vi "Test Filtering.vi"(8 "error in (no error)":errorcluster) -> (0 "error out":errorcluster)   [LabVIEW 2020]
uses:
  a02d23f6-73dd-4d4c-9f99-b180725647c3.vi
  533fd5d0-9135-456a-82c4-707cf62dfcc0.vi
  b2c899c7-82cb-45de-b54c-0f6bbd6c2dd8.vi
  1299700a-be9c-46a6-9b80-003b6c5b12f7.vi
  808b52e7-524e-4250-8ad6-d26fecc8b44a.vi
  3354226a-df3f-4c2f-8e3d-1360450e1ad8.vi
  205459d0-1598-4474-bf47-9f69c46f8ece.vi
  486e4e40-c95f-4fac-875a-f5feb60e7227.vi
  533fd5d0-9135-456a-82c4-707cf62dfcc0.vi/44d2b068-fa24-42c4-b7ce-acd781796053.vi
  533fd5d0-9135-456a-82c4-707cf62dfcc0.vi/f7e9a4a8-169a-4713-a4c5-2a646feda0be.vi
  533fd5d0-9135-456a-82c4-707cf62dfcc0.vi/4f5c7ada-fea6-4248-8bb4-58b212ee00ca.vi
  b2c899c7-82cb-45de-b54c-0f6bbd6c2dd8.vi/d1fab985-9124-480e-b8bc-aa5377d2de92.vi
  1299700a-be9c-46a6-9b80-003b6c5b12f7.vi/b73cea84-e472-4b9c-965d-660adbe74b39.vi
  808b52e7-524e-4250-8ad6-d26fecc8b44a.vi/683d2099-e00c-4551-b026-3c1073bcb77e.vi
  3354226a-df3f-4c2f-8e3d-1360450e1ad8.vi/eacad6df-34c9-4c9e-8205-0119b8e818d4.vi
  205459d0-1598-4474-bf47-9f69c46f8ece.vi/8ef18e61-07fd-42c8-9af4-61308265cf71.vi
  205459d0-1598-4474-bf47-9f69c46f8ece.vi/8f8b69a5-3137-4430-b83e-41fe2cca619b.vi
  205459d0-1598-4474-bf47-9f69c46f8ece.vi/2a0a81ed-9654-4ad9-8980-5ddc2610bcd7.vi
  205459d0-1598-4474-bf47-9f69c46f8ece.vi/17cfa5ab-349d-4170-9ba1-b7281e37bcf7.vi
  486e4e40-c95f-4fac-875a-f5feb60e7227.vi/6ddd74e0-5d25-4d4f-89c3-674211749c19.vi
  486e4e40-c95f-4fac-875a-f5feb60e7227.vi/1dcbab8f-0ca2-4569-972e-ee80beb773d1.vi
  486e4e40-c95f-4fac-875a-f5feb60e7227.vi/9005e1d8-42db-4b2c-8892-941e6a8eeacc.vi
  486e4e40-c95f-4fac-875a-f5feb60e7227.vi/8a9e105b-ea02-4efd-9282-f92cd78db5c5.vi
  b2c899c7-82cb-45de-b54c-0f6bbd6c2dd8.vi/d1fab985-9124-480e-b8bc-aa5377d2de92.vi/eacad6df-34c9-4c9e-8205-0119b8e818d4.vi
  486e4e40-c95f-4fac-875a-f5feb60e7227.vi/8a9e105b-ea02-4efd-9282-f92cd78db5c5.vi/8aece534-05e1-49aa-ae6d-ba885b1b7e2e.vi
  <vilib>/addons/_JKI Toolkits/Caraya/classes/Assert/Assert Equal Value and Type_Variant.vi
  <vilib>/addons/_JKI Toolkits/Caraya/classes/Assert/Assert Equal Value_Variant.vi
  <vilib>/Comparison/Equal/Equal Functor/Equal Functor.lvclass
  <vilib>/addons/_JKI Toolkits/Caraya/classes/Test/Test.lvclass
  <vilib>/addons/_JKI Toolkits/Caraya/classes/Assert/Assert.lvclass
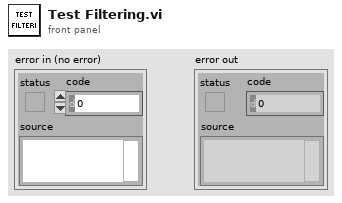
[diagram p1: front panel]
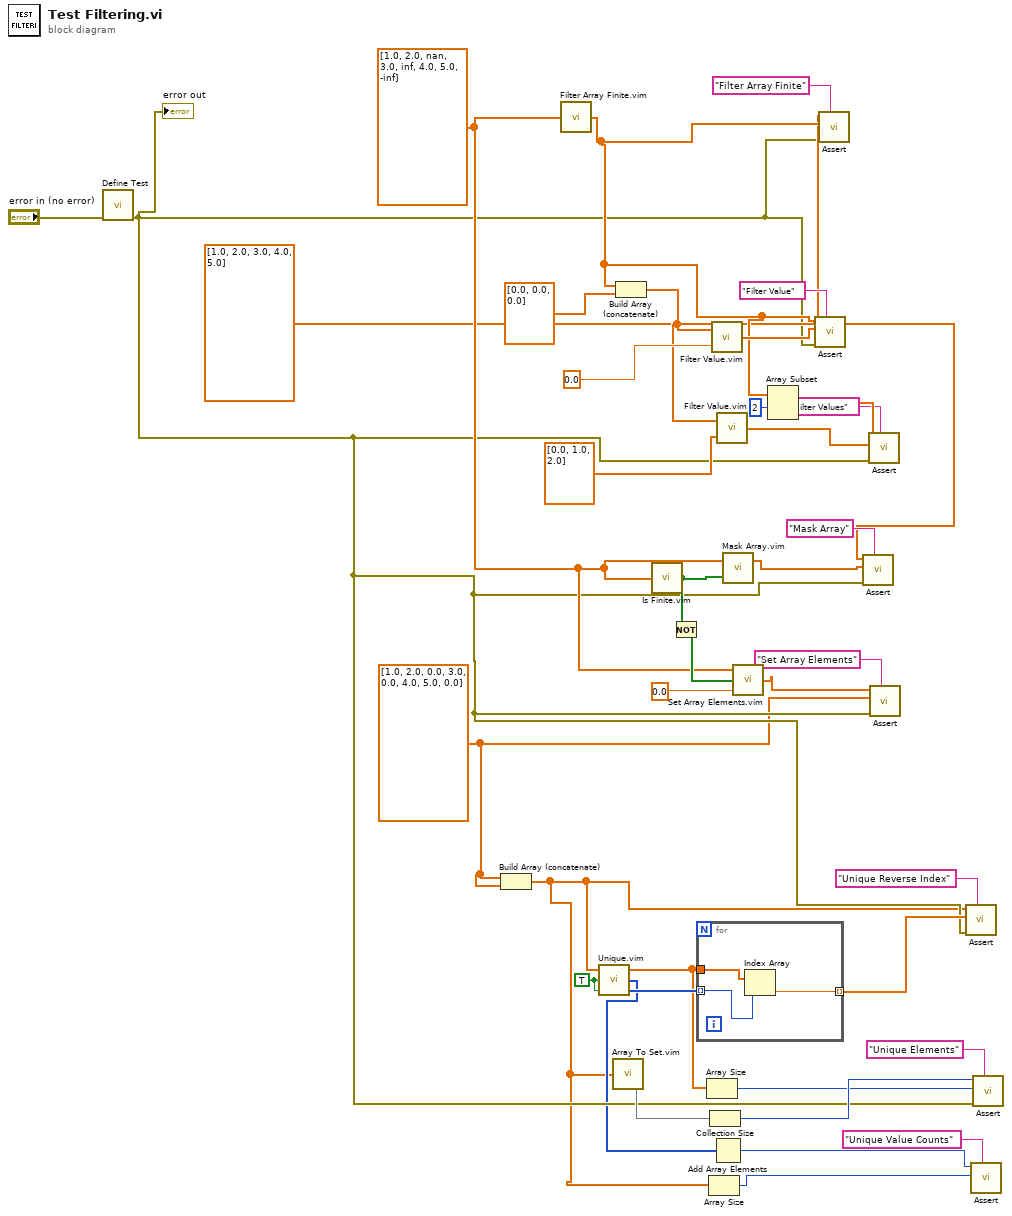
[diagram p0: block diagram]
diagram:
  w1 = TRUE ("Return Counts (T)")
  w6 = dbl[] [1.0, 2.0, 0.0, 3.0, 0.0, 4.0, 5.0, 0.0]
  w17 = dbl[] [1.0, 2.0, 3.0, 4.0, 5.0]
  w18 = dbl[] [1.0, 2.0, nan, 3.0, inf, 4.0, 5.0, -inf]
  n1 = call <vilib>:"Define Test.vi"("error in (no error)"="error in (no error)") -> ("error out"=w8:errorcluster)  [unwired: 10 in]
  "error out" <- w8
  n2 = Build Array (concatenate)(w6, w6) -> (w5:dbl[])
  n3 = call "Filter Array Finite.vim"("Array in"=w18) -> ("Array out"=w26:dbl[])  [unwired: 4 in]
  n4 = call "Unique.vim"("Return Rev. Indices (T)"=w1, "Return Counts (T)"=w1, "ND Array"=w5) -> ("Indices"=w16:i32[], "Counts"=w7:u64[], "Unique Elements"=w11:dbl[])
  n5 = call "Array To Set.vim"("Array"=w5) -> ("set"=w13:set{dbl})
  n6 = Build Array (concatenate)(w26, dbl[] [0.0, 0.0, 0.0] ("element")) -> (w32:dbl[])
  n7 = call "Is Finite.vim"("number(s) in"=w18) -> ("Number finite"=w23:bool[])
  n8 = Not(x=w23) -> (.not. x?=w19:bool[])
  n9 = for {
    tunnel: w11 -> [w41]
    tunnel: w16 -> [w40] mode=indexing
    tunnel: [w39] -> w15 mode=indexing
    n10 = Index Array(array=w41, index=w40) -> (element=w39:dbl)
  }
  n11 = Array Size(array=w11) -> (size(s)=w10:i32)
  n12 = Array Size(array=w5) -> (size(s)=w3:i32)
  n13 = Collection Size(1:w13) -> (0:w12:i32)
  n14 = call "Filter Value.vim"("Element(s)"=0.0, "Array"=w32) -> ("Filtered Array"=w33:dbl[])  [unwired: 1 in]
  n15 = Add Array Elements(numeric array=w7) -> (sum=w4:u64)
  n16 = call "Filter Value.vim"("Element(s)"=dbl[] [0.0, 1.0, 2.0], "Array"=w32) -> ("Filtered Array"=w30:dbl[])  [unwired: 1 in]
  n17 = call "Mask Array.vim"("Mask"=w23, "Array"=w18) -> ("Masked Array"=w25:dbl[])  [unwired: 1 out]
  n18 = call "Set Array Elements.vim"("Value"=0.0, "Mask"=w19, "Array"=w18) -> ("Modified Array"=w21:dbl[])
  n19 = Array Subset(array=w26, index=2) -> (w28:dbl[])  [unwired: 1 in]
  n20 = call-poly <vilib>:"Assert.vi"("Label"="Filter Value", "error in (no error)"=w8, "Y"=w33, "X"=w26) -> ()  [unwired: 7 in, 1 out]
  n21 = call-poly <vilib>:"Assert.vi"("Label"="Filter Array Finite", "error in (no error)"=w8, "Y"=w26, "X"=w17) -> ()  [unwired: 7 in, 1 out]
  n22 = call-poly <vilib>:"Assert.vi"("Label"="Mask Array", "error in (no error)"=w8, "Y"=w25, "X"=w17) -> ()  [unwired: 7 in, 1 out]
  n23 = call-poly <vilib>:"Assert.vi"("Label"="Filter Values", "error in (no error)"=w8, "Y"=w30, "X"=w28) -> ()  [unwired: 7 in, 1 out]
  n24 = call-poly <vilib>:"Assert.vi"("Label"="Set Array Elements", "error in (no error)"=w8, "Y"=w6, "X"=w21) -> ()  [unwired: 7 in, 1 out]
  n25 = call-poly <vilib>:"Assert.vi"("Label"="Unique Reverse Index", "error in (no error)"=w8, "Y"=w15, "X"=w5) -> ()  [unwired: 7 in, 1 out]
  n26 = call-poly <vilib>:"Assert.vi"("Label"="Unique Value Counts", "Y"=w3, "X"=w4) -> ()  [unwired: 8 in, 1 out]
  n27 = call-poly <vilib>:"Assert.vi"("Label"="Unique Elements", "error in (no error)"=w8, "Y"=w10, "X"=w12) -> ()  [unwired: 7 in, 1 out]
